vi "Read Sum.vi"(11 "TestActor in":refnum<class "TestActor2.lvclass">) -> (2 "Sum":dbl, 3 "TestActor out":refnum<class "TestActor2.lvclass">)   [LabVIEW 2011, in "TestActor2.lvclass"]
uses:
  TestActor2.lvclass
  TestActor2.lvclass/TestActor2.ctl
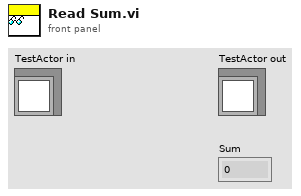
[diagram p1: front panel]
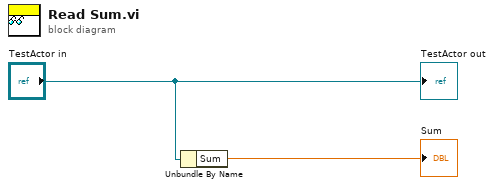
[diagram p0: block diagram]
diagram:
  n1 = Unbundle By Name("TestActor in") -> ("Sum"=→"Sum":dbl)
  "TestActor out" <- "TestActor in"
